vi "Request API.vi"(7 "API Type":refnum<class "API.lvclass">, 8 "error in (no error)":errorcluster, 11 "EnQr":refnum<class "Message Enqueuer.lvclass">) -> (0 "error out":errorcluster, 2 "API":refnum<class "API.lvclass">)   [LabVIEW 2020, in "Volatus.lvlib"]
uses:
  Volatus.lvlib
  <vilib>/ActorFramework/Message Enqueuer/Message Enqueuer.lvclass
  API/API.lvclass
  ApiValue/ApiValue.lvclass
  C:/dev/lv20CE/relink/lv-promises/Promises/Value/Value.lvclass
  lv-promises/Promises/Promise/Promise.lvclass/Promise.ctl
  lv-promises/Promises/Future/Future.lvclass/Future.ctl
  API Provider Messages/Request API Msg/Request API Msg.lvclass/Request API Msg.ctl
  <vilib>/ActorFramework/Message Enqueuer/Message Enqueuer.lvclass/Message Enqueuer.ctl
  <vilib>/ActorFramework/Message Enqueuer/Enqueue.vi
  API Provider Messages/Request API Msg/Request API Msg.lvclass
  C:/Program Files (x86)/National Instruments/LabVIEW 2020/vi.lib/ActorFramework/Message/Message.lvclass
  <vilib>/ActorFramework/Message Priority Queue/Priority Enqueue.vi
  lv-promises/Promises/Future/Future.lvclass
  lv-promises/Promises/Promise/Promise.lvclass
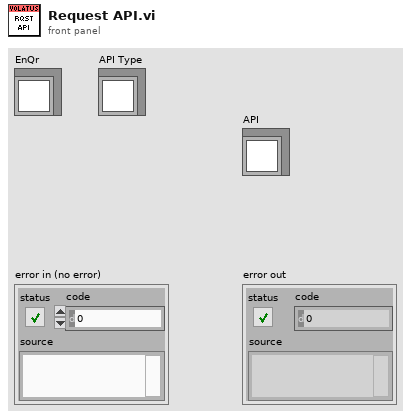
[diagram p1: front panel]
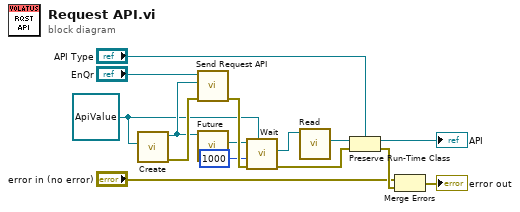
[diagram p0: block diagram]
diagram:
  w10 = refnum<class "ApiValue.lvclass"> refnum ("Volatus:ApiValue.lvclass")
  n1 = call "Create.vi"("Result Type"=w10) -> ("error out"=w13:errorcluster, "Promise"=w12:refnum<class "Promise.lvclass">)  [unwired: 9 in]
  n2 = call "Send Request API.vi"("error in (no error)"=w13, "Promise"=w12, "Message Enqueuer"="EnQr") -> ("error out"=w15:errorcluster)  [unwired: 7 in, 1 out]
  n3 = call "Future.vi"("Promise in"=w12) -> ("Future"=w11:refnum<class "Future.lvclass">)  [unwired: 9 in, 1 out]
  n4 = call "Wait.vi"("Result Type"=w10, "error in (no error)"=w15, "Timeout mS (-1)"=1000, "Future in"=w11) -> ("error out"=w6:errorcluster, "Result"=w8:refnum<class "ApiValue.lvclass">)  [unwired: 6 in]
  n5 = call "Read.vi"("ApiValue in"=w8) -> ("API"=w7:refnum<class "API.lvclass">)  [unwired: 10 in]
  n6 = Preserve Run-Time Class(object in=w7, error in=w6, 2:"API Type") -> (object out=→"API":refnum<class "API.lvclass">, error out=w3:errorcluster)
  n7 = Merge Errors("error in (no error)", w3) -> (→"error out":errorcluster)
